vi "Stop Core.vi"(10 "final error code":i32, 11 "Cooler Controller in":refnum<class "Cooler Controller.lvclass">) -> (3 "Cooler Controller out":refnum<class "Cooler Controller.lvclass">)   [LabVIEW 2025, in "Cooler Controller.lvlib" / "Cooler Controller.lvclass"]
doc: "In override VIs of Stop Core.vi, an actor should invoke any code needed to stop all the parallel processes that it created during its run. This includes any nested actors that it created and any other asynchronously running VIs, such as a Time-Delayed Message. It may also include all parallel loops in its Actor Core, although it is acceptable to stop those using a local signal on the Actor Core block diagram that is raised after the Call Parent Node finishes. \n\nThe <b>final error code</b> input tells the actor what error was set when this actor quit. Zero means there was no error. You can use this to decide whether this should be treated as a Normal Stop or an Emergency Stop for the purposes of signaling other actors. In general, any non-zero value should be treated as an Emergency Stop, though a given actor is free to choose other policies. Note that the particular error code 1608 indicates that this actor was itself stopped by an Emergency Stop and should pass that along."
uses:
  Cooler Controller.lvclass
  Cooler Controller.lvclass/Cooler Controller.ctl
  <vilib>/ActorFramework/Stop Msg/Stop Msg.lvclass/Stop Msg.ctl
  <vilib>/ActorFramework/Message Enqueuer/Message Enqueuer.lvclass/Message Enqueuer.ctl
  <vilib>/ActorFramework/Message Enqueuer/Enqueue Critical.vi
  <vilib>/ActorFramework/Stop Msg/Stop Msg.lvclass
  C:/Program Files/National Instruments/LabVIEW 2025/vi.lib/ActorFramework/Message/Message.lvclass
  <vilib>/ActorFramework/Message Priority Queue/Priority Enqueue.vi
  <vilib>/ActorFramework/Actor/Actor.lvclass
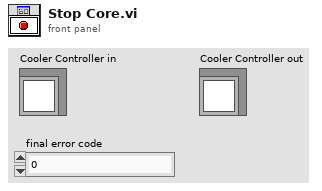
[diagram p1: front panel]
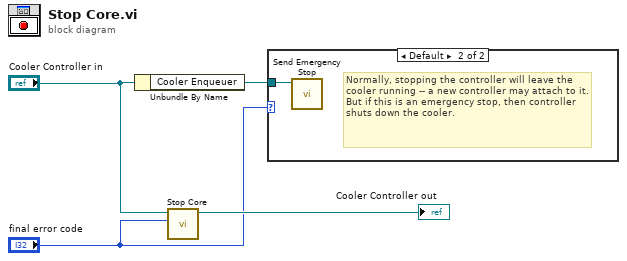
[diagram p0: block diagram]
diagram:
  n1 = Unbundle By Name("Cooler Controller in") -> ("Cooler Enqueuer"=w3:refnum<class "Message Enqueuer.lvclass">)
  n2 = call-parent "Stop Core.vi"("final error code"="final error code", "Actor in"="Cooler Controller in") -> ("Actor out"=→"Cooler Controller out":refnum<class "Cooler Controller.lvclass">)  [unwired: 9 in]
  n3 = case shown="Default" "final error code" {
    tunnel: w3 -> [_ w5]
    frame 0 {
      # "Normal stop leaves cooler running."
    }
    frame Default {
      # "Normally, stopping the controller will leave the cooler running -- a new controller may attach to it. But if this is an emergency stop, then controller shuts down the cooler."
      n4 = call <vilib>:"Send Emergency Stop.vi"("Message Enqueuer"=w5) -> ()  [unwired: 10 in, 1 out]
    }
  }
